vi "Identify.vi"(8 "error in (no error)":errorcluster, 11 "NF in":refnum<class "NF.lvclass">) -> (0 "error out":errorcluster, 2 "Plugin is Valid":bool, 3 "NF out":refnum<class "NF.lvclass">)   [LabVIEW 2018, in "NF.lvlib" / "NF.lvclass"]
uses:
  NF.lvclass
  C:/Sequence Automation/Plugins/Measurement Interface.lvlibp/Measurement Interface.lvclass
  Plugins/Measurement Interface.lvlibp/Private Methods/Measurement Definition Entry/Read Measurement Definition Entry.vi
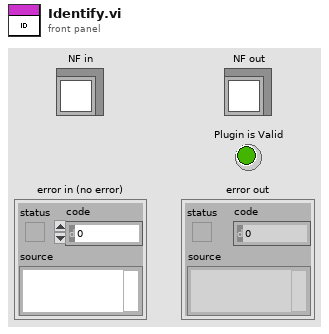
[diagram p1: front panel]
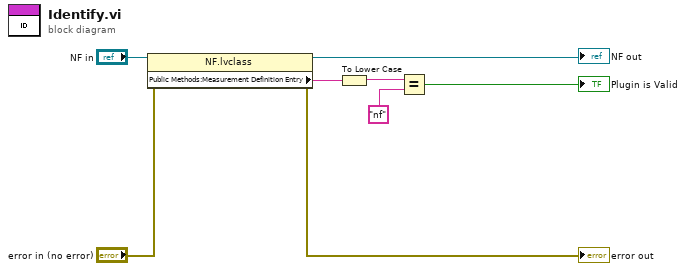
[diagram p0: block diagram]
diagram:
  n1 = property class="NF.lvclass"(reference="NF in", error in="error in (no error)") -> (reference out=→"NF out":refnum<class "NF.lvclass">, error out=→"error out":errorcluster, "Public Methods:Measurement Definition Entry"=w6:string)
  n2 = To Lower Case(string=w6) -> (all lower case string=w5:string)
  n3 = Equal?(x=w5, y="nf") -> (x = y?=→"Plugin is Valid":bool)
